vi "undo.vi"(8 "error in (no error)":errorcluster, 11 "ScriptEditorV2 in":refnum<class "ScriptEditorV2.lvclass">) -> (0 "error out":errorcluster, 3 "ScriptEditorV2 out":refnum<class "ScriptEditorV2.lvclass">)   [LabVIEW 2009, in "Views.lvlib" / "ScriptEditor.lvlib" / "ScriptEditorV2.lvclass"]
uses:
  ScriptEditorV2.lvclass
  ScriptEditorV2.lvclass/ScriptEditorV2.ctl
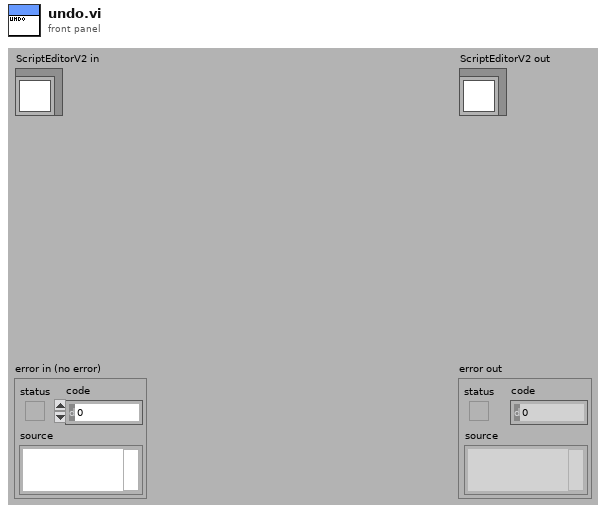
[diagram p1: front panel]
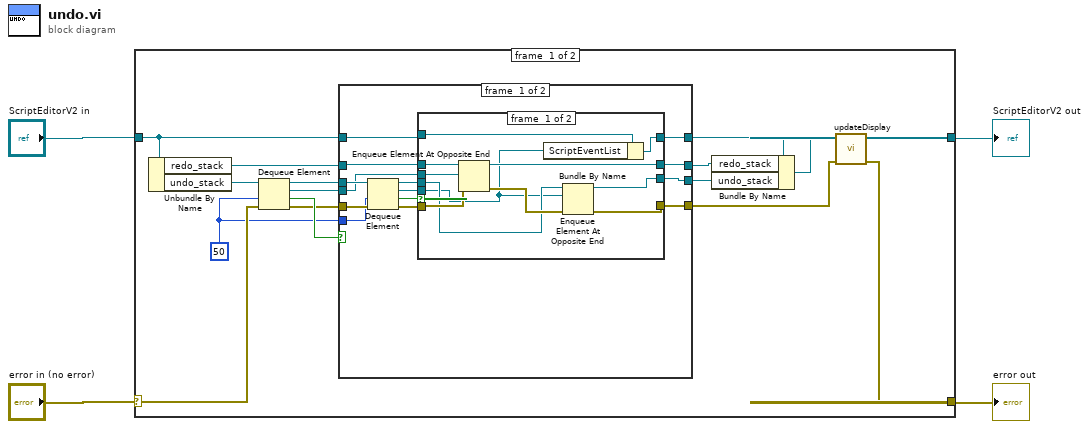
[diagram p0: block diagram]
diagram:
  n1 = case shown="No Error" "error in (no error)" {
    selector: "error in (no error)" -> [w19 w55]
    tunnel: [w5 w55] -> w3
    tunnel: [w7 w54] -> w1
    tunnel: "ScriptEditorV2 in" -> [w17 w54]
    frame #0 {
      w9 = 50
      n2 = Unbundle By Name(w17) -> ("redo_stack"=w16:refnum<queue>, "undo_stack"=w20:refnum<queue>)
      n3 = Dequeue Element(queue=w20, timeout in ms (-1)=w9, error in (no error)=w19) -> (queue out=w15:refnum<queue>, element=w11:refnum<class "ScriptEventList.lvclass">, timed out?=w18:bool, error out=w10:errorcluster)
      n4 = case shown="False" w18 {
        tunnel: w17 -> [w34 w53]
        tunnel: w16 -> [w25 w51]
        tunnel: [w33 w53] -> w13
        tunnel: w15 -> [w32 w52]
        tunnel: [w23 w52] -> w14
        tunnel: [w22 w51] -> w12
        tunnel: w11 -> [w27 _]
        tunnel: w10 -> [w31 w50]
        tunnel: w9 -> [w29 _]
        tunnel: [w21 w50] -> w6
        frame #0 {
          n5 = Dequeue Element(queue=w32, timeout in ms (-1)=w29, error in (no error)=w31) -> (queue out=w26:refnum<queue>, element=w28:refnum<class "ScriptEventList.lvclass">, timed out?=w30:bool, error out=w24:errorcluster)
          n6 = case shown="False" w30 {
            tunnel: w34 -> [w45 w49]
            tunnel: [w44 w49] -> w33
            tunnel: w28 -> [w36 _]
            tunnel: w27 -> [w42 _]
            tunnel: w26 -> [w38 w48]
            tunnel: w25 -> [w43 w47]
            tunnel: w24 -> [w41 w46]
            tunnel: [w37 w48] -> w23
            tunnel: [w40 w47] -> w22
            tunnel: [w35 w46] -> w21
            frame #0 {
              n7 = Enqueue Element At Opposite End(queue=w43, element=w42, error in (no error)=w41) -> (queue out=w40:refnum<queue>, error out=w39:errorcluster)  [unwired: 1 in, 1 out]
              n8 = Bundle By Name(cluster=w45, "ScriptEventList"=w36) -> (w44:refnum<class "ScriptEditorV2.lvclass">)
              n9 = Enqueue Element At Opposite End(queue=w38, element=w36, error in (no error)=w39) -> (queue out=w37:refnum<queue>, error out=w35:errorcluster)  [unwired: 1 in, 1 out]
            }
            frame #1 {
            }
          }
        }
        frame #1 {
          # "timeout"
        }
      }
      n10 = Bundle By Name(cluster=w13, "redo_stack"=w12, "undo_stack"=w14) -> (w8:refnum<class "ScriptEditorV2.lvclass">)
      n11 = call "updateDisplay.vi"("error in (no error)"=w6, "ScriptEditorV2 in"=w8) -> ("error out"=w5:errorcluster, "ScriptEditorV2 out"=w7:refnum<class "ScriptEditorV2.lvclass">)  [unwired: 8 in]
    }
    frame #1 {
    }
  }
  "error out" <- w3
  "ScriptEditorV2 out" <- w1
